vi "Handle Error.vi"(8 "error in (no error)":errorcluster, 11 "Error Enqueuer in":refnum<user-event>) -> (0 "error out":errorcluster, 3 "Error Enqueuer out":refnum<user-event>)   [LabVIEW 2018, in "Scripting.lvlib" / "Actor.lvclass"]
uses:
  Actor.lvclass
  <vilib>/event_ctls.llb/usereventprio.ctl
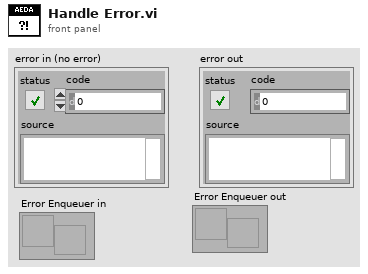
[diagram p1: front panel]
types:
  T1 = typedef "usereventprio.ctl" = enum32{"high priority", "normal priority"}
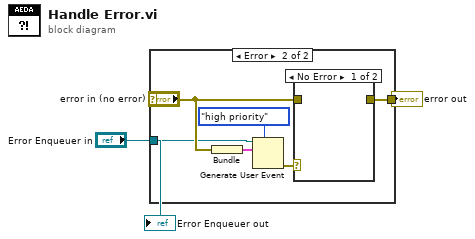
[diagram p0: block diagram]
diagram:
  n1 = case shown="Error" "error in (no error)" {
    selector: "error in (no error)" -> [w4 w7]
    tunnel: [w4 w9] -> w3
    tunnel: "Error Enqueuer in" -> [_ w5]
    frame No Error {
    }
    frame Error {
      n2 = Bundle("error IO"=w7) -> (w6:cluster{"error IO":errorcluster})  [unwired: 1 in]
      n3 = Generate User Event(priority (normal)=usereventprio."high priority", user event=w5, event data cluster=w6) -> (error out=w10:errorcluster)  [unwired: 1 in, 1 out]
      n4 = case shown="No Error" w10 {
        tunnel: [_ w11] -> w9
        tunnel: w7 -> [_ w11]
        frame No Error {
        }
        frame Error {
        }
      }
    }
  }
  "error out" <- w3
  "Error Enqueuer out" <- "Error Enqueuer in"
